vi "mean.vi"(8 "error in (no error)":errorcluster, 11 "PositionSignals in":refnum<class "PositionSignals.lvclass">) -> (0 "error out":errorcluster, 1 "standard deviation (x/y/z)":dbl[][](array[numeric]), 2 "mean (x/y/z)":dbl[][](array[numeric]), 3 "PositionSignals out":refnum<class "PositionSignals.lvclass">)   [LabVIEW 2010, in "PositionSignals.lvclass"]
uses:
  PositionSignals.lvclass
  PositionSignals.lvclass/PositionSignals.ctl
  common/classes/ImageCollection/ImageCollection/add_mode_enum.ctl
  common/classes/ImageCollection/ImageCollection/ImageCollection.lvclass
  common/classes/Image/Image/Image.lvclass
  <vilib>/Analysis/NI_AALBase.lvlib
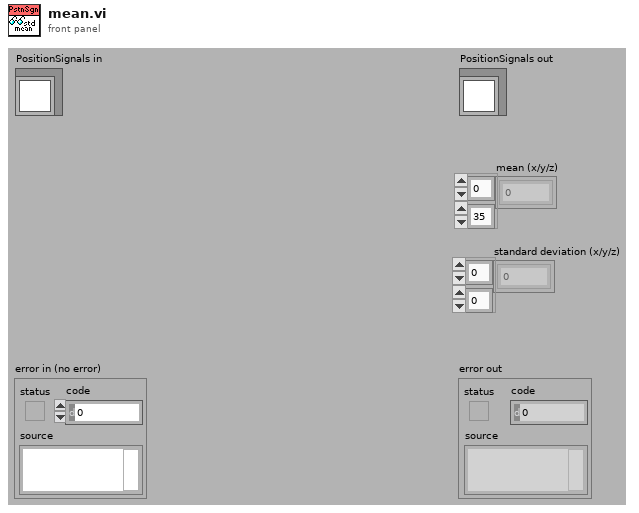
[diagram p1: front panel]
types:
  T1 = typedef "ImageCollection.lvclass/add_mode_enum.ctl" = enum16{"instance", "copy"}
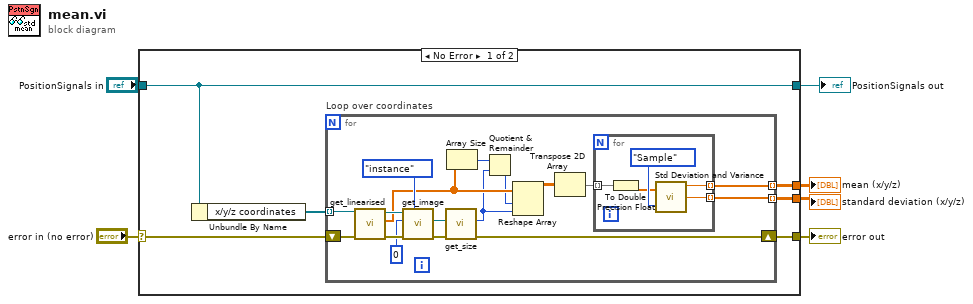
[diagram p0: block diagram]
diagram:
  n1 = case shown="No Error" "error in (no error)" {
    selector: "error in (no error)" -> [w11 w36]
    tunnel: [w10 w36] -> w5
    tunnel: [w12 w35] -> w3
    tunnel: "PositionSignals in" -> [w12 w35]
    tunnel: [w8 _] -> w2
    tunnel: [w7 _] -> w1
    frame No Error {
      n2 = Unbundle By Name(w12) -> ("x/y/z coordinates"=w9:refnum<class "ImageCollection.lvclass">[])
      n3 = for "Loop over coordinates" {
        shift-right: [w20] -> w10
        shift-left: w11 -> [w29]
        tunnel: w9 -> [w28] mode=indexing
        tunnel: [w23] -> w7 mode=indexing
        tunnel: [w18] -> w8 mode=indexing
        n4 = call "get_linearised.vi"("error in (no error)"=w29, "ImageCollection in"=w28) -> ("error out"=w25:errorcluster, "pixels"=w17:sgl[], "ImageCollection out"=w24:refnum<class "ImageCollection.lvclass">)  [unwired: 7 in]
        n5 = call-dynamic "get_image.vi"("get image as..."=add_mode_enum."instance", "error in (no error)"=w25, "index"=0, "ImageCollection in"=w24) -> ("error out"=w26:errorcluster, "Image.lvclass"=w27:refnum<class "Image.lvclass">)  [unwired: 5 in, 1 out]
        n6 = call-dynamic "get_size.vi"("error in (no error)"=w26, "Image in"=w27) -> ("error out"=w20:errorcluster, "x resolution"=w16:i32)  [unwired: 2 in, 6 out]
        n7 = Array Size(array=w17) -> (size(s)=w19:i32)
        n8 = Quotient & Remainder(x=w19, y=w16) -> (floor(x/y)=w15:i32)  [unwired: 1 out]
        n9 = Reshape Array(w17, w15, w16) -> (w14:sgl[][])
        n10 = Transpose 2D Array(2D array=w14) -> (transposed array=w13:sgl[][])
        n11 = for {
          tunnel: w13 -> [w34] mode=indexing
          tunnel: [w33] -> w18 mode=indexing
          tunnel: [w31] -> w23 mode=indexing
          n12 = To Double Precision Float(number=w34) -> (double precision float=w30:dbl[])
          n13 = call <vilib>:"Std Deviation and Variance.vi"("X"=w30, "Weighting (Sample)"=enum16{"Sample", "Population"}."Sample") -> ("mean"=w33:dbl, "standard deviation"=w31:dbl)  [unwired: 1 out]
        }
      }
    }
    frame Error {
    }
  }
  "error out" <- w5
  "PositionSignals out" <- w3
  "mean (x/y/z)" <- w2
  "standard deviation (x/y/z)" <- w1
